vi "GDSLvClass_GetRootBaseClass.vi"(0 "ViRef/Path,LvClassRef/Path":variant, 5 "error in (no error)":errorcluster, 6 "Don'tOpenReference":bool, 7 "LimitToSpecificProviderTypeOfSameType(True)":bool=TRUE) -> (13 "RootClassVersion":string, 14 "RootBaseClassRef":refnum<vi>, 15 "RootBaseClassPath":path, 16 "ClassName":string, 17 "InheritanceHierarchy":T1[](array[typedef]), 18 "Qualified Class Name":string, 19 "error out":errorcluster)   [LabVIEW 2020]
uses:
  <resource>/Framework/Providers/Open_GDS/ClassProviders/Common/LvClass_class/GDSLvClass_ClassInfo.ctl
  <resource>/Framework/Providers/Open_GDS/ClassProviders/Provider_EndevoGOOP300/ClassWriterGOOP300_class/ClassWriterGOOP300.lvclass
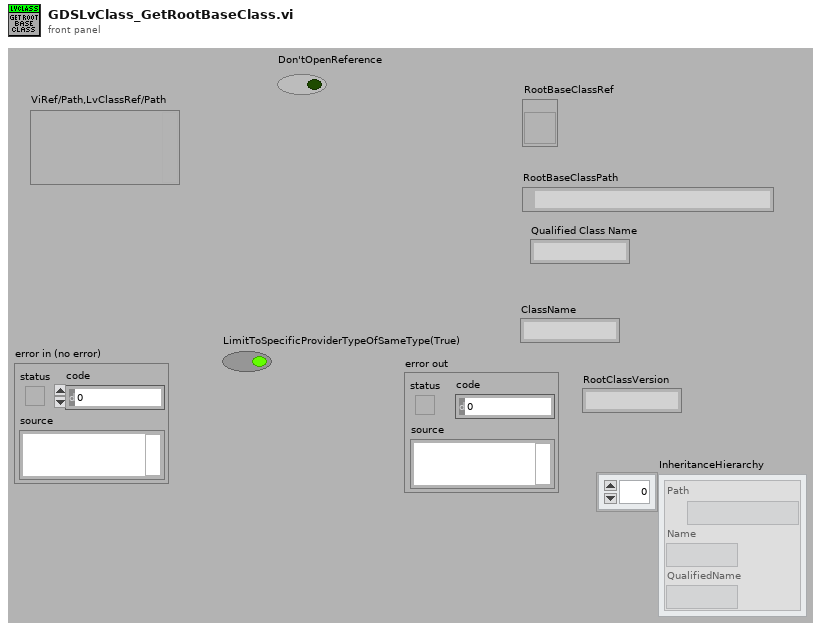
[diagram p1: front panel]
types:
  T1 = typedef "GDSLvClass_ClassInfo.ctl" = cluster{"Path":path, "Name":string, "QualifiedName":string}
  T2 = typedef "GDSLvCLass_ClassSettingsType.ctl" = cluster{"ClassProviderName":string, "ClassTemplateUsed":string, "ClassTemplateVersion":string, "ClassDescription":string, "PlugIns":T3[], "ConnectorPanePattern":string}
  T3 = typedef "GDSLvClass_PlugIn.ctl" = cluster{"Type":T4, "ID":string, "Version":string, "Path":path, "Name":string, "Data":variant}
  T4 = typedef "GDSLvClass_PlugInTypes.ctl" = enum16{"DesignPattern", "MethodTypes"}
  T5 = cluster{"Major":u16, "Minor":u16, "Fix":u16, "Build":u16}
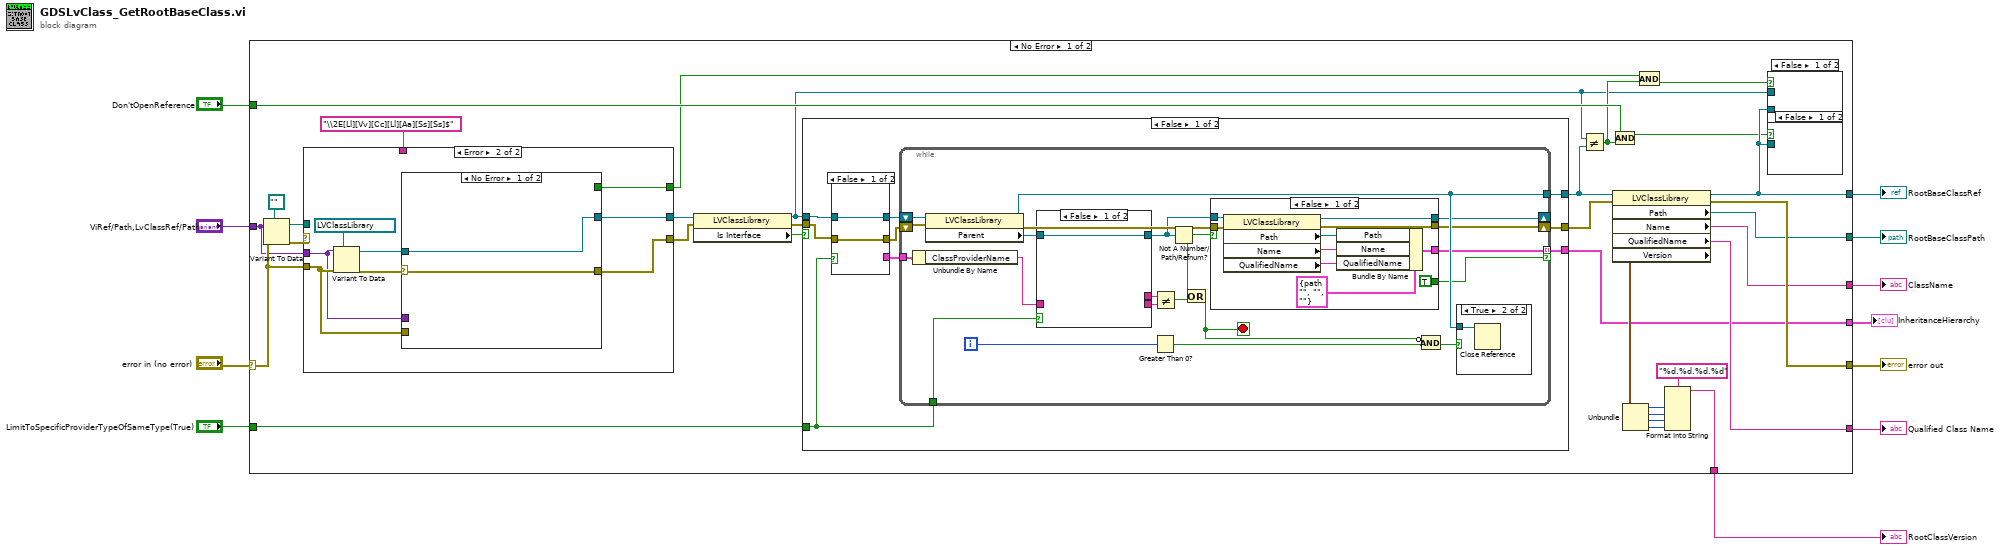
[diagram p0: block diagram]
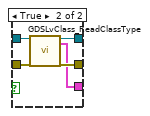
[diagram p2: hidden frame]
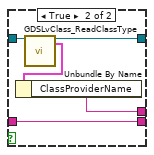
[diagram p4: hidden frame]
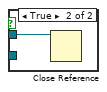
[diagram p7: hidden frame]
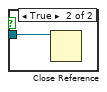
[diagram p8: hidden frame]
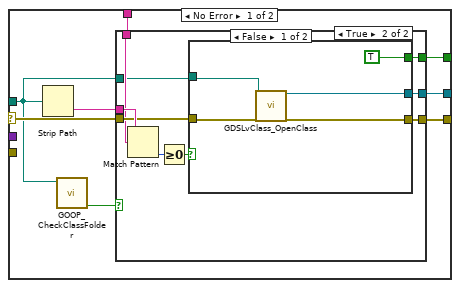
[diagram p9: hidden frame]
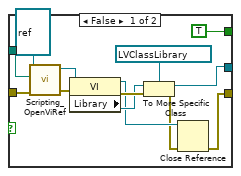
[diagram p10: hidden frame]
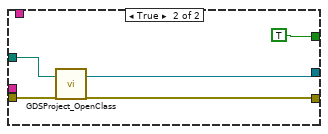
[diagram p11: hidden frame]
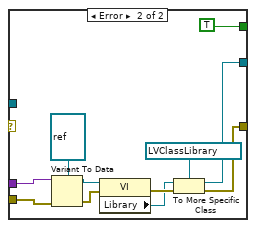
[diagram p12: hidden frame]
diagram:
  n1 = case shown="No Error" "error in (no error)" {
    selector: "error in (no error)" -> [w37 w165]
    tunnel: "ViRef/Path,LvClassRef/Path" -> [w36 _]
    tunnel: [w39 w165] -> w10
    tunnel: [w33 _] -> w8
    tunnel: [w38 _] -> w7
    tunnel: "Don'tOpenReference" -> [w34 _]
    tunnel: [w28 _] -> w5
    tunnel: "LimitToSpecificProviderTypeOfSameType(True)" -> [w26 _]
    tunnel: [w25 _] -> w3
    tunnel: [w18 _] -> w2
    tunnel: [w12 _] -> w1
    frame No Error {
      n2 = Variant To Data(error in=w37, type=path "", Variant=w36) -> (data=w41:path, error out=w42:errorcluster)
      n3 = case shown="Error" w42 {
        selector: w42 -> [w110 _]
        tunnel: w41 -> [w105 _]
        tunnel: [w109 w146] -> w16
        tunnel: [w108 w147] -> w17
        tunnel: w37 -> [_ w150]
        tunnel: w36 -> [_ w145]
        tunnel: [w107 w144] -> w31
        tunnel: "\\2E[Ll][Vv][Cc][Ll][Aa][Ss][Ss]$" ("regular expression") -> [w106 _]
        frame No Error {
          n4 = Strip Path(path=w105) -> (name=w111:string)  [unwired: 1 out]
          n5 = call <resource>:"GOOP_CheckClassFolder.vi"("Class Or Class Floder"=w105) -> ("ClassFolder"=w104:bool)  [unwired: 6 in, 4 out]
          n6 = case shown="False" w104 {
            tunnel: w111 -> [w120 _]
            tunnel: w110 -> [w118 w142]
            tunnel: [w116 w141] -> w109
            tunnel: [w115 w140] -> w108
            tunnel: [w114 TRUE] -> w107
            tunnel: w106 -> [w113 _]
            tunnel: w105 -> [w112 w143]
            frame False {
              n7 = Match Pattern(string=w120, regular expression=w113) -> (offset past match=w119:i32)  [unwired: 1 in, 3 out]
              n8 = Greater Or Equal To 0?(x=w119) -> (x >= 0?=w117:bool)
              n9 = case shown="True" w117 {
                tunnel: w112 -> [w132 w138]
                tunnel: w118 -> [w133 w137]
                tunnel: [w123 w136] -> w116
                tunnel: [w126 w135] -> w115
                tunnel: [TRUE TRUE] -> w114
                frame False {
                  n10 = call <resource>:"Scripting_OpenViRef.vi"("error in"=w133, "ViPath/ViName/Viref"=w132, "AppRef"=refnum<vi> refnum) -> ("error out"=w131:errorcluster, "vi reference"=w130:refnum<vi>)  [unwired: 6 in, 1 out]
                  n11 = property class="VI"(reference=w130, error in=w131) -> (reference out=w125:refnum<vi>, error out=w129:errorcluster, "Library"=w128:refnum<vi>)
                  n12 = To More Specific Class(target class=refnum<vi> refnum ("LVClass.Open"), reference=w128, error in=w129) -> (specific class reference=w126:refnum<vi>, error out=w124:errorcluster)
                  n13 = Close Reference(reference=w125, error in (no error)=w124) -> (error out=w123:errorcluster)
                }
                frame True {
                  n14 = call <resource>:"GDSLvClass_OpenClass.vi"("ClassToOpen"=w138, "error in (no error)"=w137) -> ("LVClass.Open"=w135:refnum<vi>, "error out"=w136:errorcluster)  [unwired: 16 in]
                }
              }
            }
            frame True {
              n15 = call <resource>:"GDSProject_OpenClass.vi"("ClassPath(FilePath/ProjectTreePath/LvCLassRef)"=w143, "error IO"=w142) -> ("LVClass.Open"=w140:refnum<vi>, "error out"=w141:errorcluster)  [unwired: 15 in, 1 out]
            }
          }
        }
        frame Error {
          n16 = Variant To Data(error in=w150, type=refnum<vi> refnum ("LVClass.Open"), Variant=w145) -> (data=w148:refnum<vi>, error out=w149:errorcluster)
          n17 = case shown="No Error" w149 {
            selector: w149 -> [w152 _]
            tunnel: w150 -> [_ w163]
            tunnel: w148 -> [w153 _]
            tunnel: [w153 w156] -> w147
            tunnel: [w152 w155] -> w146
            tunnel: w145 -> [_ w162]
            tunnel: [_ TRUE] -> w144
            frame No Error {
            }
            frame Error {
              n18 = Variant To Data(error in=w163, type=refnum<vi> refnum ("vi reference"), Variant=w162) -> (data=w157:refnum<vi>, error out=w158:errorcluster)
              n19 = property class="VI"(reference=w157, error in=w158) -> (error out=w161:errorcluster, "Library"=w160:refnum<vi>)  [unwired: 1 out]
              n20 = To More Specific Class(target class=refnum<vi> refnum ("LVClass.Open"), reference=w160, error in=w161) -> (specific class reference=w156:refnum<vi>, error out=w155:errorcluster)
            }
          }
        }
      }
      n21 = property class="LVClassLibrary"(reference=w17, error in=w16) -> (reference out=w13:refnum<vi>, error out=w15:errorcluster, "Is Interface"=w14:bool)
      n22 = case shown="False" w14 {
        tunnel: [w52 w101] -> w40
        tunnel: [w51 w100] -> w35
        tunnel: w26 -> [w48 _]
        tunnel: w13 -> [w46 w100]
        tunnel: w15 -> [w45 w101]
        tunnel: [w44 _] -> w12
        frame False {
          n23 = case shown="False" w48 {
            tunnel: w46 -> [w54 w59]
            tunnel: w45 -> [w53 w58]
            tunnel: [w54 w57] -> w50
            tunnel: [w53 w56] -> w49
            tunnel: [_ w55] -> w47
            frame False {
            }
            frame True {
              n24 = call <resource>:"GDSLvClass_ReadClassType.vi"("Class Refnum In"=w59, "error in (no error)"=w58) -> ("Class Refnum Out"=w57:refnum<vi>, "ClassSettings"=w55:T2, "error out"=w56:errorcluster)  [unwired: 15 in]
            }
          }
          n25 = while {
            shift-right: [w64] -> _
            shift-left: w50 -> [w80]
            tunnel: [w78] -> w51
            shift-right: [w65] -> w52
            shift-left: w49 -> [w79]
            tunnel: w48 -> [w74]
            tunnel: w47 -> [w70]
            tunnel: [w61] -> w44 mode=indexing if=w60
            i -> [w76]
            stop <- w62 stop-if-true
            n26 = Unbundle By Name(w70) -> ("ClassProviderName"=w69:string)
            n27 = property class="LVClassLibrary"(reference=w80, error in=w79) -> (reference out=w78:refnum<vi>, error out=w67:errorcluster, "Parent"=w73:refnum<vi>)
            n28 = case shown="False" w74 {
              tunnel: w73 -> [w93 w98]
              tunnel: [w93 w97] -> w66
              tunnel: [_ w95] -> w72
              tunnel: w69 -> [_ w94]
              tunnel: [_ w94] -> w71
              frame False {
              }
              frame True {
                n29 = call <resource>:"GDSLvClass_ReadClassType.vi"("Class Refnum In"=w98) -> ("Class Refnum Out"=w97:refnum<vi>, "ClassSettings"=w96:T2)  [unwired: 16 in, 1 out]
                n30 = Unbundle By Name(w96) -> ("ClassProviderName"=w95:string)
              }
            }
            n31 = Greater Than 0?(x=w76) -> (x > 0?=w75:bool)
            n32 = Not Equal?(x=w72, y=w71) -> (x != y?=w68:bool)
            n33 = Not A Number/Path/Refnum?(number/path/refnum=w66) -> (NaN/Path/Refnum?=w63:bool)
            n34 = Or(x=w63, y=w68) -> (x .or. y?=w62:bool)
            n35 = case shown="False" w63 {
              tunnel: w67 -> [w90 w91]
              tunnel: w66 -> [w89 w92]
              tunnel: [w88 w91] -> w65
              tunnel: [w87 w92] -> w64
              tunnel: [w82 _] -> w61
              tunnel: [TRUE _] -> w60
              frame False {
                n36 = property class="LVClassLibrary"(reference=w89, error in=w90) -> (reference out=w87:refnum<vi>, error out=w88:errorcluster, "Path"=w85:path, "Name"=w84:string, "QualifiedName"=w83:string)
                n37 = Bundle By Name(cluster=T1 {"Path"=path "", "Name"="", "QualifiedName"=""} ("ClassInfo"), "Path"=w85, "Name"=w84, "QualifiedName"=w83) -> (w82:T1)
              }
              frame True {
              }
            }
            n38 = Compound Arithmetic op=AND(invert w62, w75) -> (w77:bool)
            n39 = case shown="True" w77 {
              tunnel: w78 -> [_ w99]
              frame False {
              }
              frame True {
                n40 = Close Reference(reference=w99) -> ()  [unwired: 1 in, 1 out]
              }
            }
          }
        }
        frame True {
        }
      }
      n41 = Not Equal?(x=w13, y=w35) -> (x != y?=w29:bool)
      n42 = property class="LVClassLibrary"(reference=w35, error in=w40) -> (reference out=w33:refnum<vi>, error out=w39:errorcluster, "Path"=w38:path, "Name"=w28:string, "QualifiedName"=w25:string, "Version"=w19:T5)
      n43 = Compound Arithmetic op=AND(w34, w29) -> (w32:bool)
      n44 = Unbundle(w19) -> ("Major"=w23:u16, "Minor"=w22:u16, "Fix"=w21:u16, "Build"=w20:u16)
      n45 = Compound Arithmetic op=AND(w31, w29) -> (w30:bool)
      n46 = Format Into String(format string="%d.%d.%d.%d", w23, w22, w21, w20) -> (resulting string=w18:string)  [unwired: 2 in, 1 out]
      n47 = case shown="False" w30 {
        tunnel: w13 -> [_ w102]
        tunnel: w33 -> [_ _]
        frame False {
        }
        frame True {
          n48 = Close Reference(reference=w102) -> ()  [unwired: 1 in, 1 out]
        }
      }
      n49 = case shown="False" w32 {
        tunnel: w33 -> [_ w103]
        frame False {
        }
        frame True {
          n50 = Close Reference(reference=w103) -> ()  [unwired: 1 in, 1 out]
        }
      }
    }
    frame Error {
    }
  }
  "RootBaseClassRef" <- w8
  "RootBaseClassPath" <- w7
  "error out" <- w10
  "ClassName" <- w5
  "Qualified Class Name" <- w3
  "RootClassVersion" <- w2
  "InheritanceHierarchy" <- w1
